vi "Msg.vi"(7 "Actor in":refnum<class "Actor.lvclass">, 11 "Finish Msg in":refnum<class "Finish Msg.lvclass">) -> (0 "Error out":errorcluster, 5 "Actor out":refnum<class "Actor.lvclass">)   [LabVIEW 2025, in "jettl.lvlib" / "Finish Msg.lvlib" / "Finish Msg.lvclass"]
uses:
  Finish Msg.lvclass
  Actor/Actor/Actor.lvclass
  Finish/Finish.lvclass
  Finish Msg.lvclass/Finish Msg.ctl
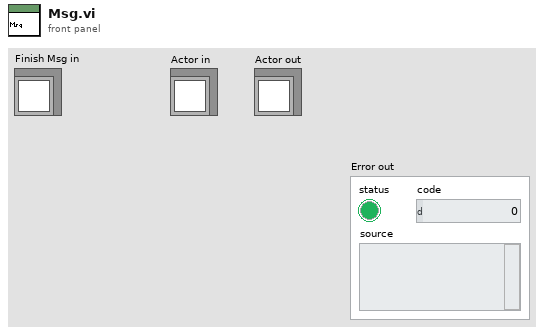
[diagram p1: front panel]
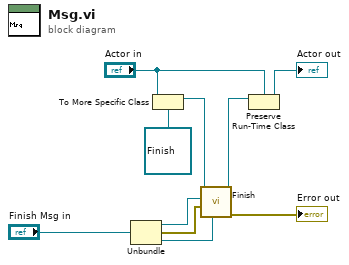
[diagram p0: block diagram]
diagram:
  n1 = Unbundle "Unbundle"("Finish Msg in") -> (w3:refnum<class "Actor.lvclass">, w2:errorcluster, w1:refnum<class "Sender.lvclass">)
  n2 = To More Specific Class(target class=refnum<class "Finish.lvclass"> refnum ("jettl.lvlib:jettl Msg Last Ack Creator Queue.lvlib:jettl Msg Last Ack Creator Queue.lvclass"), reference="Actor in") -> (specific class reference=w6:refnum<class "Finish.lvclass">)  [unwired: 1 in, 1 out]
  n3 = call-dynamic "Finish.vi"("Sender"=w1, "Error"=w2, "Actor"=w3, "Finish in"=w6) -> ("Error out"=→"Error out":errorcluster, "Finish out"=w5:refnum<class "Finish.lvclass">)  [unwired: 6 in]
  n4 = Preserve Run-Time Class(object in=w5, 2:"Actor in") -> (object out=→"Actor out":refnum<class "Actor.lvclass">)  [unwired: 1 in, 1 out]
